vi "ReadOrWriteToJSONfile.vi"(7 "Data":T1, 8 "error in (no error)":errorcluster, 10 "Command":enum16{"Read", "Write"}(ring), 11 "JSONtext Input":string) -> (0 "error out":errorcluster, 3 "JSON text":string)   [LabVIEW 2017]
doc: "<B>This VI is used for Read or Write a JSON file.</B>"
uses:
  <vilib>/JDP Science/JSONtext/JSONtext.lvlib
  Ctrl/Property.ctl
  Ctrl/PhysicalChannel.ctl
  Ctrl/Bitfield.ctl
  Ctrl/Register.ctl
  Ctrl/ScaleType.ctl
  Ctrl/Scale.ctl
  Ctrl/EnumValue.ctl
  Ctrl/Enum.ctl
  Ctrl/Caps.ctl
  Ctrl/Data.ctl
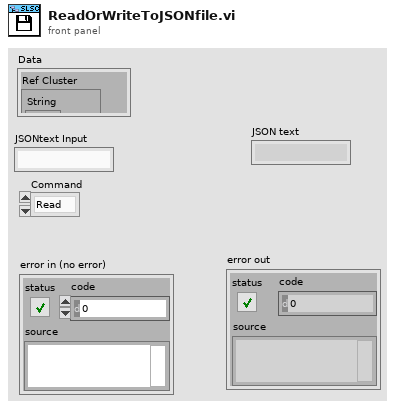
[diagram p1: front panel]
types:
  T1 = typedef "Data.ctl" = cluster{"Ref Cluster":cluster{"String":refnum<vi>, "U8":refnum<vi>, "I8":refnum<vi>, "U32":refnum<vi>, "I32":refnum<vi>, "U64":refnum<vi>, "I64":refnum<vi>, "Ring":refnum<vi>, "DBL":refnum<vi>, "Add":refnum<vi>, "Remove":refnum<vi>, "Property tree":refnum<vi>, "confirm":refnum<vi>}, "JSON Text":string, "Original JSON Text":string, "Caps":T2, "SLSC Output Tree":cluster{"Left Cell String":string, "Child Text":string[], "Child Tag":string, "Item Indent":i32, "Child Only?":bool, "Glyph Index":i32, "offline value":variant}[], "Ref Index and Control Type":cluster{"index":i32, "Datatype":string}, "Selected Type and name":cluster{"Selected Type":enum16{"Property", "Physical Channel", "Other"}, "Selected Property Name":string}, "Update whole Tree?":bool}
  T2 = typedef "Caps.ctl" = cluster{"properties":T3[], "physical channels":T4[], "registers":T5[], "scales":T7[], "enums":T9[], "productName":string}
  T3 = typedef "Property.ctl" = cluster{"name":string, "bitfield":string, "value":variant, "dataType":string, "min":variant, "max":variant, "scale":string, "access":string}
  T4 = typedef "PhysicalChannel.ctl" = cluster{"name":string, "properties":T3[]}
  T5 = typedef "Register.ctl" = cluster{"name":string, "address":i32, "size":i32, "bitfields":T6[], "initialValue":variant, "connectedProperties":string[]}
  T6 = typedef "Bitfield.ctl" = cluster{"name":string, "offset":i32, "size":i32, "signed":bool}
  T7 = typedef "Scale.ctl" = cluster{"name":string, "type":T8, "params":variant}
  T8 = typedef "ScaleType.ctl" = enum16{"NoScale", "Table", "Polynomial", "Linear"}
  T9 = typedef "Enum.ctl" = cluster{"name":string, "values":T10[]}
  T10 = typedef "EnumValue.ctl" = cluster{"name":string, "value":i32}
  T11 = enum16{"open", "replace", "create", "open or create", "replace or create", "replace or create with confirmation"}
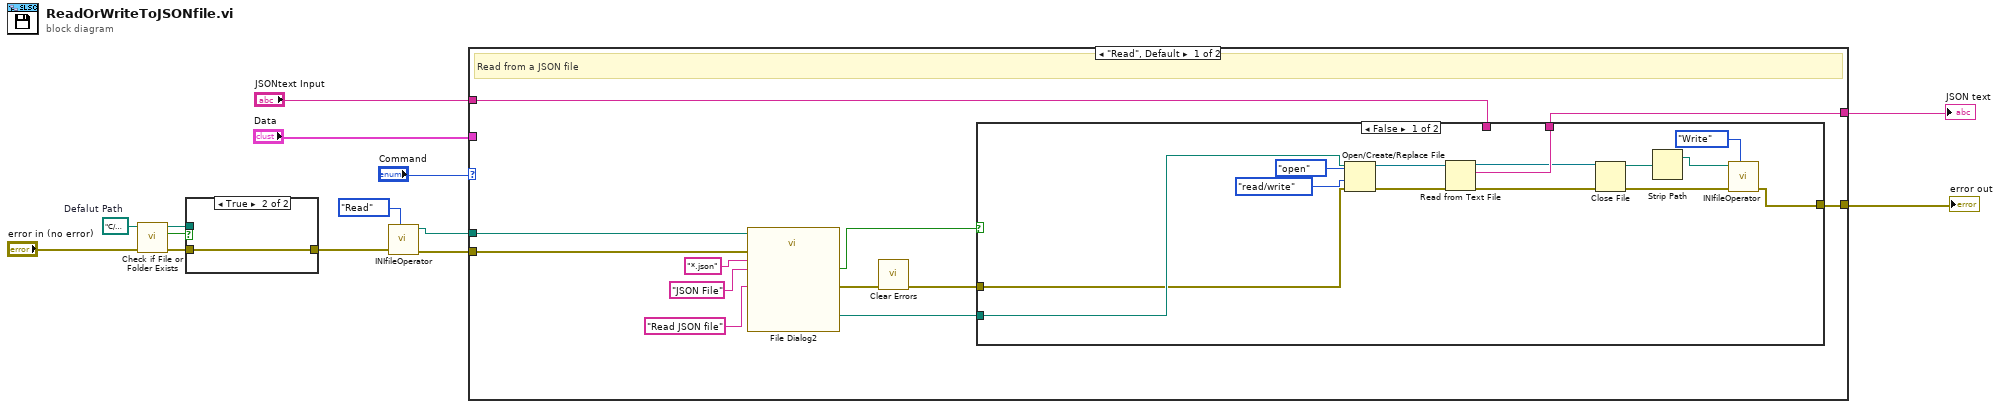
[diagram p0: block diagram]
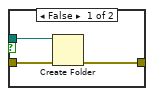
[diagram p2: hidden frame]
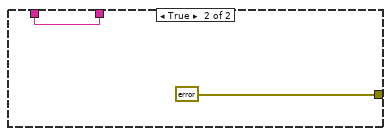
[diagram p3: hidden frame]
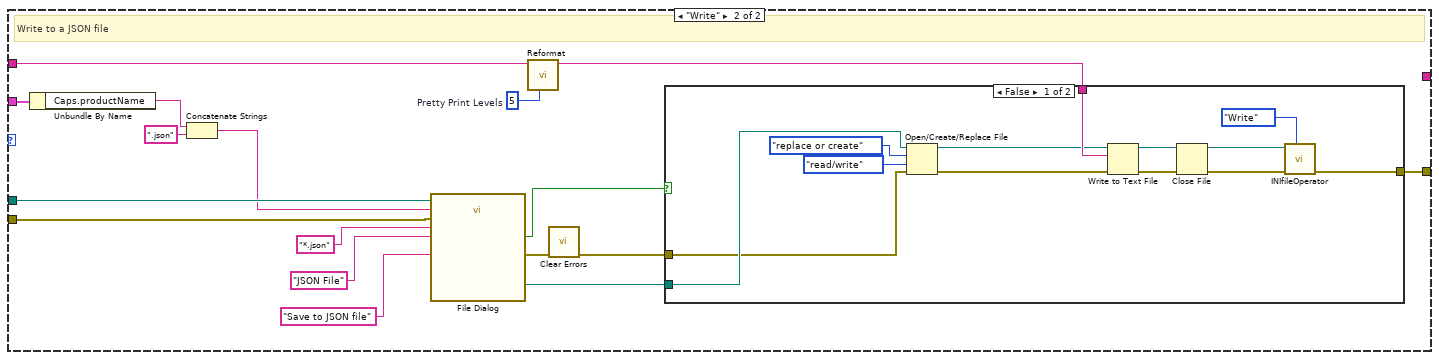
[diagram p4: hidden frame]
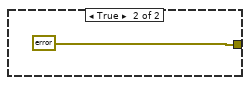
[diagram p5: hidden frame]
diagram:
  w6 = path "C:/ProgramData/National Instruments/nislsc/capabilities"  # Defalut Path
  n1 = call <vilib>:"Check if File or Folder Exists.vi"("error in (no error)"="error in (no error)", "path"=w6) -> ("error out"=w4:errorcluster, "file or folder exists?"=w5:bool, "dup path"=w3:path)  [unwired: 7 in]
  n2 = case shown="True" w5 {
    tunnel: w4 -> [w17 w18]
    tunnel: w3 -> [w16 _]
    tunnel: [w15 w18] -> w1
    frame False {
      n3 = Create Folder(path (use dialog)=w16, error in=w17) -> (error out=w15:errorcluster)  [unwired: 1 in, 2 out]
    }
    frame True {
    }
  }
  n4 = call "INIfileOperator.vi"("Command"=enum16{"Write", "Read"}."Read", "error in (no error)"=w1) -> ("error out"=w8:errorcluster, "Last Path output"=w7:path)  [unwired: 8 in]
  n5 = case shown="\"Read\", Default" "Command" {
    tunnel: "JSONtext Input" -> [w21 w49]
    tunnel: w7 -> [w29 w60]
    tunnel: w8 -> [w20 w58]
    tunnel: [w30 _] -> w14
    tunnel: [w22 w54] -> w13
    tunnel: "Data" -> [_ w53]
    frame "Read", Default {
      # "Read from a JSON file"
      n6 = call "File Dialog2"("start path"=w29, "prompt"="Read JSON file", "error in"=w20, "pattern (all files)"="*.json", "pattern label"="JSON File") -> ("selected path"=w19:path, "cancelled"=w23:bool, "error out"=w25:errorcluster)  [unwired: 7 in, 1 out]
      n7 = call <vilib>:"Clear Errors.vi"("error in (no error)"=w25) -> ("error out"=w24:errorcluster)  [unwired: 5 in, 1 out]
      n8 = case shown="False" w23 {
        tunnel: [w40 w45] -> w30
        tunnel: w19 -> [w39 _]
        tunnel: w24 -> [w38 _]
        tunnel: [w31 errorcluster {"status"=FALSE, "code"=0, "source"=""} ("error out")] -> w22
        tunnel: w21 -> [_ w45]
        frame False {
          n9 = Open/Create/Replace File(file path (use dialog)=w39, error in=w38, operation (0:open)=T11."open", access (0:read/write)=enum16{"read/write", "read-only", "write-only"}."read/write") -> (refnum out=w41:refnum<file>, error out=w42:errorcluster)  [unwired: 2 in, 1 out]
          n10 = Read from Text File(file (use dialog)=w41, error in=w42) -> (refnum out=w36:refnum<file>, text=w40:string, error out=w37:errorcluster)  [unwired: 2 in, 1 out]
          n11 = Close File(refnum=w36, error in=w37) -> (path=w34:path, error out=w35:errorcluster)
          n12 = Strip Path(path=w34) -> (stripped path=w33:path)  [unwired: 1 out]
          n13 = call "INIfileOperator.vi"("Command"=enum16{"Write", "Read", "Write Default Path"}."Write", "error in (no error)"=w35, "Last Path"=w33) -> ("error out"=w31:errorcluster)  [unwired: 7 in, 1 out]
        }
        frame True {
        }
      }
    }
    frame "Write" {
      w47 = 5  # Pretty Print Levels
      # "Write to a JSON file"
      n14 = Unbundle By Name(w53) -> ("Caps.productName"=w52:string)
      n15 = Concatenate Strings(w52, ".json" ("string")) -> (w50:string)
      n16 = call "File Dialog"("start path"=w60, "prompt"="Save to JSON file", "default name"=w50, "error in"=w58, "pattern (all files)"="*.json", "pattern label"="JSON File") -> ("selected path"=w59:path, "cancelled"=w55:bool, "error out"=w57:errorcluster)  [unwired: 6 in, 1 out]
      n17 = call <vilib>:"Reformat.vi"("Pretty Print Levels"=w47, "JSON"=w49) -> ("<JSON>First JSON Value\n\n<JSON>"=w48:string)  [unwired: 6 in, 3 out]
      n18 = call <vilib>:"Clear Errors.vi"("error in (no error)"=w57) -> ("error out"=w56:errorcluster)  [unwired: 5 in, 1 out]
      n19 = case shown="False" w55 {
        tunnel: w48 -> [w76 _]
        tunnel: w59 -> [w71 _]
        tunnel: w56 -> [w70 _]
        tunnel: [w66 errorcluster {"status"=FALSE, "code"=0, "source"=""} ("error out")] -> w54
        frame False {
          n20 = Open/Create/Replace File(file path (use dialog)=w71, error in=w70, operation (0:open)=T11."replace or create", access (0:read/write)=enum16{"read/write", "read-only", "write-only"}."read/write") -> (refnum out=w73:refnum<file>, error out=w72:errorcluster)  [unwired: 2 in, 1 out]
          n21 = Write to Text File(file (use dialog)=w73, text=w76, error in=w72) -> (refnum out=w69:refnum<file>, error out=w68:errorcluster)  [unwired: 1 in, 1 out]
          n22 = Close File(refnum=w69, error in=w68) -> (path=w65:path, error out=w67:errorcluster)
          n23 = call "INIfileOperator.vi"("Command"=enum16{"Write", "Read"}."Write", "error in (no error)"=w67, "Last Path"=w65) -> ("error out"=w66:errorcluster)  [unwired: 7 in, 1 out]
        }
        frame True {
        }
      }
    }
  }
  "error out" <- w13
  "JSON text" <- w14
